vi "Set EPI Aperture Stop.vi"(8 "error in (no error)":errorcluster {"code" format="%.0x"}, 9 "Driving Address (0)":i32, 10 "Device Number (1)":i32=1, 11 "VISA Resource Name":refnum<visa-resource-name>) -> (0 "error out":errorcluster {"code" format="%.0x"}, 3 "VISA Resource Name Out":refnum<visa-resource-name>)   [LabVIEW 2018, in "Olympus IX BX Series.lvlib"]
doc: "Specifies the diameter of EPI AS (RLAA).\n\nNotes:\n(1) This VI is valid only for Olympus BX2A model."
uses:
  Olympus IX BX Series.lvlib
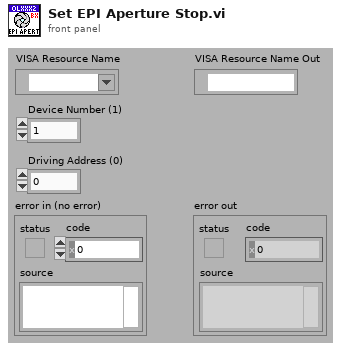
[diagram p1: front panel]
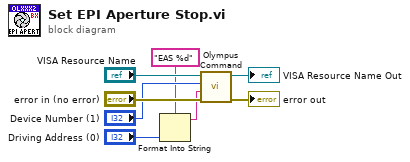
[diagram p0: block diagram]
diagram:
  n1 = Format Into String(format string="EAS %d", "Driving Address (0)") -> (resulting string=w5:string)  [unwired: 2 in, 1 out]
  n2 = call "Olympus Command.vi"("error in (no error)"="error in (no error)", "Command string"=w5, "Device Number (1)"="Device Number (1)", "VISA Resource Name"="VISA Resource Name") -> ("error out"=→"error out":errorcluster, "VISA Resource Name Out"=→"VISA Resource Name Out":refnum<visa-resource-name>)  [unwired: 5 in, 1 out]
